vi "Test Set Subpanels-- SMO Array -- Not Started.vi"(8 "error in":errorcluster) -> (0 "error out":errorcluster)   [LabVIEW 2020]
uses:
  <vilib>/JKI/JKI SMO/SMO/Typedefs/SMOState --Enum.ctl
  Maui 2.0/Maui 2.0.lvclass
  C:/Program Files (x86)/National Instruments/LabVIEW 2020/vi.lib/JKI/JKI SMO/SMO/SMO.lvclass
  <vilib>/addons/_JKI Toolkits/Caraya/classes/Assert/Assert True.vi
  <vilib>/addons/_JKI Toolkits/Caraya/classes/Assert/Assert Equal Value_Variant.vi
  <vilib>/addons/_JKI Toolkits/Caraya/classes/Test/Test.lvclass
  <vilib>/JKI/JKI SMO/SMO/SMO.lvclass
  <vilib>/addons/_JKI Toolkits/Caraya/classes/Assert/Assert.lvclass
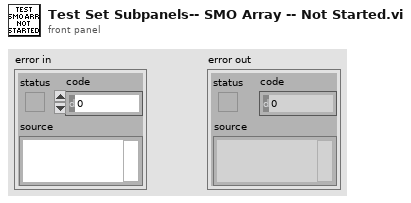
[diagram p1: front panel]
types:
  T1 = typedef "SMO.lvclass/SMOState --Enum.ctl" = enum16{"unknown", "Created", "Started", "Stopped"}
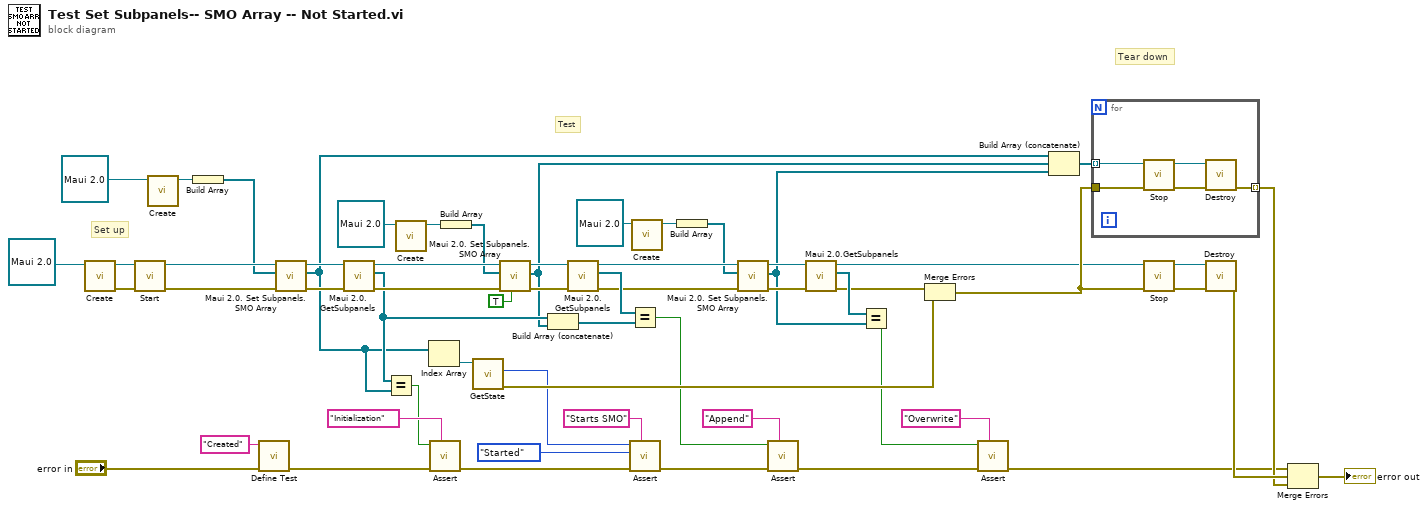
[diagram p0: block diagram]
diagram:
  # "Tear down"
  # "Test"
  # "Set up"
  n1 = call <vilib>:"Create.vi"("SMO"=refnum<class "Maui 2.0.lvclass"> refnum ("Maui 2.0.lvclass")) -> ("error out"=w56:errorcluster, "SMO out"=w55:refnum<class "Maui 2.0.lvclass">)  [unwired: 8 in, 1 out]
  n2 = call <vilib>:"Start.vi"("error in (no error)"=w56, "SMO"=w55) -> ("error out"=w53:errorcluster, "SMO out"=w52:refnum<class "Maui 2.0.lvclass">)  [unwired: 8 in]
  n3 = call <vilib>:"Create.vi"("SMO"=refnum<class "Maui 2.0.lvclass"> refnum ("Maui 2.0.lvclass")) -> ("SMO out"=w8:refnum<class "Maui 2.0.lvclass">)  [unwired: 8 in, 2 out]
  n4 = Build Array(w8) -> (w10:refnum<class "Maui 2.0.lvclass">[])
  n5 = call <vilib>:"Define Test.vi"("error in (no error)"="error in", "Label (VI Title)"="Created") -> ("error out"=w58:errorcluster)  [unwired: 9 in]
  n6 = call-dynamic "Maui 2.0. Set Subpanels.SMO Array.vi"("error in (no error)"=w53, "Subpanels"=w10, "Maui 2.0 in"=w52) -> ("error out"=w45:errorcluster, "Subpanels"=w29:refnum<class "SMO.lvclass">[], "Maui 2.0 out"=w46:refnum<class "Maui 2.0.lvclass">)  [unwired: 6 in]
  n7 = call "Maui 2.0.GetSubpanels.vi"("error in (no error)"=w45, "Maui 2.0"=w46) -> ("error out"=w31:errorcluster, "Subpanels"=w30:refnum<class "SMO.lvclass">[], "Maui 2.0 out"=w32:refnum<class "Maui 2.0.lvclass">)  [unwired: 7 in]
  n8 = Equal?(x=w30, y=w29) -> (x = y?=w28:bool)
  n9 = call <vilib>:"Create.vi"("SMO"=refnum<class "Maui 2.0.lvclass"> refnum ("Maui 2.0.lvclass")) -> ("SMO out"=w7:refnum<class "Maui 2.0.lvclass">)  [unwired: 8 in, 2 out]
  n10 = Index Array(array=w29) -> (element=w43:refnum<class "SMO.lvclass">)  [unwired: 1 in]
  n11 = call-poly <vilib>:"Assert.vi"("Label"="Initialization", "error in (no error)"=w58, "True?"=w28) -> ("error out"=w40:errorcluster)  [unwired: 8 in]
  n12 = Build Array(w7) -> (w3:refnum<class "Maui 2.0.lvclass">[])
  n13 = call <vilib>:"GetState.vi"("SMO"=w43) -> ("error out"=w39:errorcluster, "SMO State"=w12:T1)  [unwired: 8 in, 1 out]
  n14 = call-dynamic "Maui 2.0. Set Subpanels.SMO Array.vi"("Append (F)"=TRUE, "error in (no error)"=w31, "Subpanels"=w3, "Maui 2.0 in"=w32) -> ("error out"=w34:errorcluster, "Subpanels"=w24:refnum<class "SMO.lvclass">[], "Maui 2.0 out"=w33:refnum<class "Maui 2.0.lvclass">)  [unwired: 5 in]
  n15 = Build Array (concatenate)(w30, w24) -> (w26:refnum<class "SMO.lvclass">[])
  n16 = call "Maui 2.0.GetSubpanels.vi"("error in (no error)"=w34, "Maui 2.0"=w33) -> ("error out"=w20:errorcluster, "Subpanels"=w27:refnum<class "SMO.lvclass">[], "Maui 2.0 out"=w17:refnum<class "Maui 2.0.lvclass">)  [unwired: 7 in]
  n17 = Equal?(x=w27, y=w26) -> (x = y?=w11:bool)
  n18 = call-poly <vilib>:"Assert.vi"("Label"="Starts SMO", "error in (no error)"=w40, "Y"=SMOState_--Enum."Started" ("SMO State"), "X"=w12) -> ("error out"=w42:errorcluster)  [unwired: 7 in]
  n19 = call <vilib>:"Create.vi"("SMO"=refnum<class "Maui 2.0.lvclass"> refnum ("Maui 2.0.lvclass")) -> ("SMO out"=w4:refnum<class "Maui 2.0.lvclass">)  [unwired: 8 in, 2 out]
  n20 = Build Array(w4) -> (w2:refnum<class "Maui 2.0.lvclass">[])
  n21 = call-dynamic "Maui 2.0. Set Subpanels.SMO Array.vi"("error in (no error)"=w20, "Subpanels"=w2, "Maui 2.0 in"=w17) -> ("error out"=w21:errorcluster, "Subpanels"=w13:refnum<class "SMO.lvclass">[], "Maui 2.0 out"=w22:refnum<class "Maui 2.0.lvclass">)  [unwired: 6 in]
  n22 = call-poly <vilib>:"Assert.vi"("Label"="Append", "error in (no error)"=w42, "True?"=w11) -> ("error out"=w36:errorcluster)  [unwired: 8 in]
  n23 = call "Maui 2.0.GetSubpanels.vi"("error in (no error)"=w21, "Maui 2.0"=w22) -> ("error out"=w18:errorcluster, "Subpanels"=w19:refnum<class "SMO.lvclass">[], "Maui 2.0 out"=w16:refnum<class "Maui 2.0.lvclass">)  [unwired: 7 in]
  n24 = Equal?(x=w19, y=w13) -> (x = y?=w15:bool)
  n25 = Merge Errors(w18, w39) -> (w38:errorcluster)
  n26 = call-poly <vilib>:"Assert.vi"("Label"="Overwrite", "error in (no error)"=w36, "True?"=w15) -> ("error out"=w35:errorcluster)  [unwired: 8 in]
  n27 = Build Array (concatenate)(w29, w24, w13) -> (w48:refnum<class "SMO.lvclass">[])
  n28 = for {
    tunnel: w48 -> [w62] mode=indexing
    tunnel: w38 -> [w61]
    tunnel: [w60] -> w47 mode=indexing
    n29 = call <vilib>:"Stop.vi"("error in (no error)"=w61, "SMO"=w62) -> ("error out"=w63:errorcluster, "SMO out"=w64:refnum<class "SMO.lvclass">)  [unwired: 8 in]
    n30 = call <vilib>:"Destroy.vi"("error in (no error)"=w63, "SMO"=w64) -> ("error out"=w60:errorcluster)  [unwired: 9 in]
  }
  n31 = call <vilib>:"Stop.vi"("error in (no error)"=w38, "SMO"=w16) -> ("error out"=w51:errorcluster, "SMO out"=w50:refnum<class "Maui 2.0.lvclass">)  [unwired: 8 in]
  n32 = call <vilib>:"Destroy.vi"("error in (no error)"=w51, "SMO"=w50) -> ("error out"=w49:errorcluster)  [unwired: 9 in]
  n33 = Merge Errors(w35, w49, w47) -> (→"error out":errorcluster)
